vi "Initialize Listbox.vi"(8 "error in":errorcluster, 10 "Expected DevIDs":T1[](array[typedef]), 11 "MulticolumnListbox in":refnum<vi>) -> (0 "error out":errorcluster, 3 "dup MulticolumnListbox":refnum<vi>)   [LabVIEW 2018, in "EMS User Interface Actor.lvlib" / "EMS User Interface.lvclass"]
uses:
  EMS User Interface Actor/EMS User Interface/EMS User Interface.lvclass
  <vilib>/ORNL/CSEISMIC DDS/CSEISMIC DDS Base/Data Types/Controls/DeviceID.ctl
  <vilib>/Utility/miscctls.llb/LVRowAndColumnTypeDef.ctl
  <vilib>/ORNL/CSEISMIC DDS/CSEISMIC DDS Base/CSEISMIC DDS.lvclass
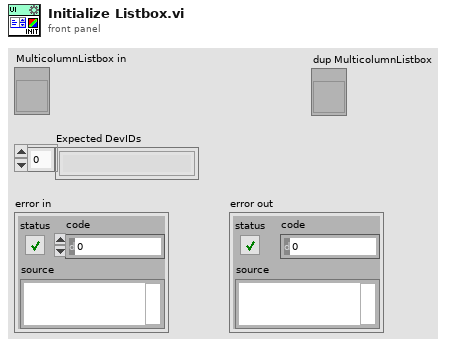
[diagram p1: front panel]
types:
  T1 = typedef "CSEISMIC DDS.lvlib/CSEISMIC DDS.lvclass/DeviceID.ctl" = string
  T2 = typedef "LVRowAndColumnTypeDef.ctl" = cluster{"Row":i32, "Column":i32}
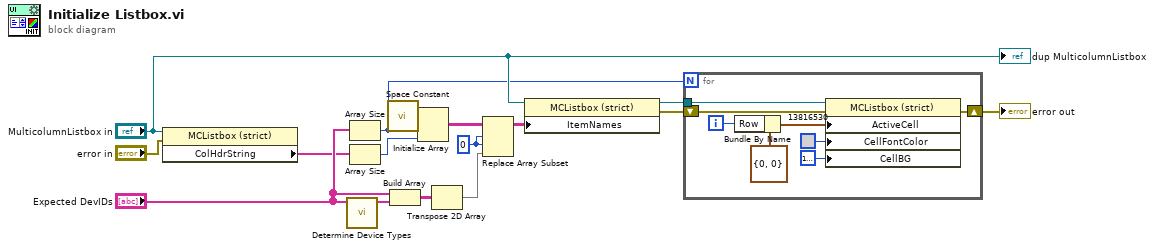
[diagram p0: block diagram]
diagram:
  w3 = 0 ("index (row)")
  n1 = property on="Property Node" class="MCListbox (strict)"(reference="MulticolumnListbox in", error in="error in") -> ("ColHdrString"=w7:string[])  [unwired: 2 out]
  n2 = call "Determine Device Types.vi"("DeviceIDs"="Expected DevIDs") -> ("Device Classes"=w12:string[])  [unwired: 9 in]
  n3 = Array Size(array="Expected DevIDs") -> (size(s)=w1:i32)
  n4 = Array Size(array=w7) -> (size(s)=w6:i32)
  n5 = call <vilib>:"Space Constant.vi"() -> ("String"=w8:string)
  n6 = Build Array("Expected DevIDs", w12) -> (w16:T1[][])
  n7 = Initialize Array(w8, w1, w6) -> (w5:string[][])
  n8 = Transpose 2D Array(2D array=w16) -> (transposed array=w2:T1[][])
  n9 = Replace Array Subset(array=w5, new element=w2, index (row)=w3, index (col)=w3) -> (w4:string[][])
  n10 = property on="Property Node" class="MCListbox (strict)"(reference="MulticolumnListbox in", "ItemNames"=w4) -> (reference out=w14:refnum<vi>, error out=w15:errorcluster)  [unwired: 1 in]
  n11 = for {
    N: w1 -> [_]
    shift-right: [w18] -> w13
    shift-left: w15 -> [w19]
    tunnel: w14 -> [w20]
    i -> [w23]
    n12 = Bundle By Name(cluster=T2 {"Row"=0, "Column"=0} ("Active Cell:Active Cell"), "Row"=w23) -> (w22:T2)
    n13 = property on="Property Node" class="MCListbox (strict)"(reference=w20, error in=w19, "ActiveCell"=w22, "CellFontColor"=u32 13816530, "CellBG"=u32 16777226) -> (error out=w18:errorcluster)  [unwired: 1 out]
  }
  "error out" <- w13
  "dup MulticolumnListbox" <- "MulticolumnListbox in"
